vi "Write Ramp Rate.vi"(8 "error in (no error)":errorcluster, 9 "Time Stamp":timestamp, 10 "Ramp Rate [degC/s]":dbl, 11 "Thermal Chamber Response Simlator In":refnum<class "Thermal Chamber Response Simlator.lvclass">) -> (0 "error out":errorcluster, 3 "Thermal Chamber Response Simlator Out":refnum<class "Thermal Chamber Response Simlator.lvclass">)   [LabVIEW 2020, in "Thermal Chamber Response Simlator.lvclass"]
uses:
  Thermal Chamber Response Simlator.lvclass
  Thermal Chamber Response Simlator.lvclass/Thermal Chamber Response Simlator.ctl
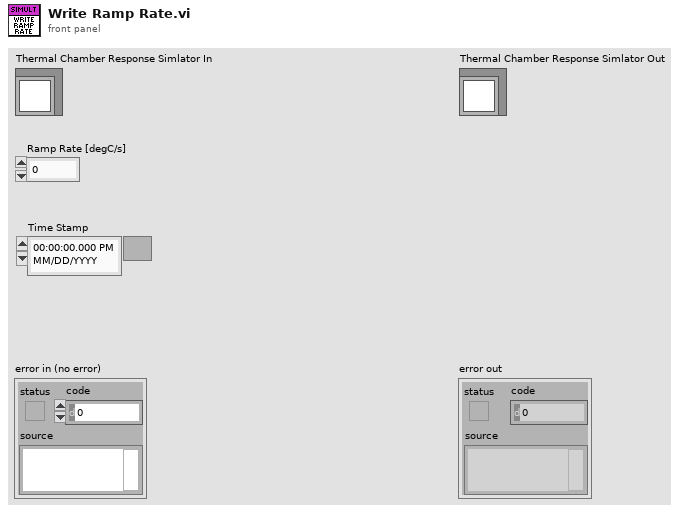
[diagram p1: front panel]
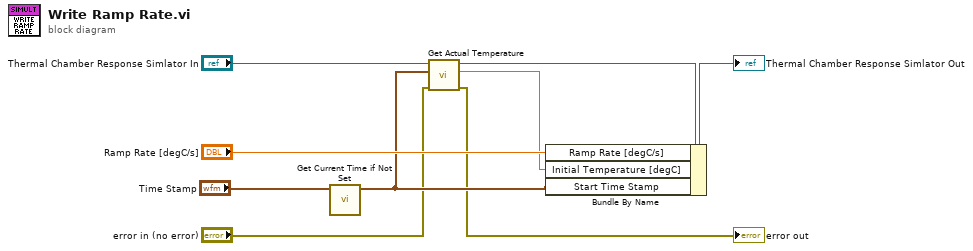
[diagram p0: block diagram]
diagram:
  n1 = call "Get Current Time if Not Set.vi"("Start Time"="Time Stamp") -> ("seconds since 1Jan1904"=w3:timestamp)  [unwired: 10 in]
  n2 = call "Get Actual Temperature.vi"("error in (no error)"="error in (no error)", "Time Stamp"=w3, "Thermal Chamber Response Simlator In"="Thermal Chamber Response Simlator In") -> ("error out"=→"error out":errorcluster, "Actual Temperature [degC]"=w4:dbl, "Thermal Chamber Response Simlator Out"=w5:refnum<class "Thermal Chamber Response Simlator.lvclass">)  [unwired: 6 in]
  n3 = Bundle By Name(cluster=w5, "Ramp Rate [degC/s]"="Ramp Rate [degC/s]", "Initial Temperature [degC]"=w4, "Start Time Stamp"=w3) -> (→"Thermal Chamber Response Simlator Out":refnum<class "Thermal Chamber Response Simlator.lvclass">)
